vi "ros_test.vi"() -> ()   [LabVIEW 2015]
uses:
  <vilib>/Tufts CEEO ROS for LabVIEW Software/ROS/Code/Console/Servers/ServerSubs/TopicDef.ctl
  <vilib>/Tufts CEEO ROS for LabVIEW Software/ROS/Code/SubVIs/_ROSDirection.ctl
  <vilib>/Tufts CEEO ROS for LabVIEW Software/ROS/MessageParsing/std_msgs/subs/parse_i32_scalar.vi
panel:
  in  "stop":bool
  out "number":i32
  in  "node":string
  in  "Definitions":T1={"Topic"="/robot/head/command_head_nod", "Type"="std_msgs/Bool", "Action"=enum."Publisher", "Update (ms)"=1, "queue size"=1}
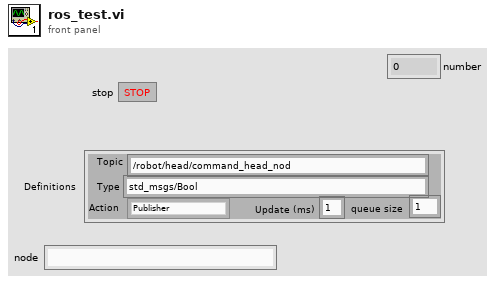
[diagram p1: front panel]
types:
  T1 = typedef "TopicDef.ctl" = cluster{"Topic":string, "Type":string, "Action":T2, "Update (ms)":u16, "queue size":u16}
  T2 = typedef "_ROSDirection.ctl" = enum16{"Node", "Publisher", "Subscriber", "ServiceClient", "ServiceProvider"}
  T3 = typedef "_ROSControl.ctl" = cluster{"topic port":u16, "Node":string, "topic":string, "type":string, "node port":u16, "error ":errorcluster, "Direction":T2, "Update (ms)":u16, "FIFO size":u16}
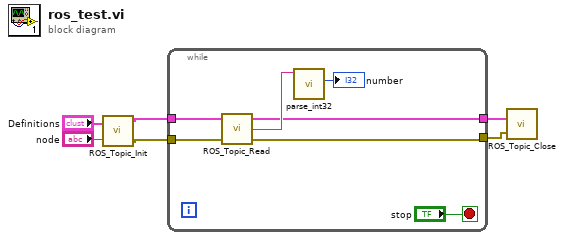
[diagram p0: block diagram]
diagram:
  n1 = call <vilib>:"ROS_Topic_Init.vi"("Definitions"="Definitions", "node"="node") -> ("ROS out"=w2:T3, "error out"=w1:errorcluster)  [unwired: 1 in]
  n2 = while {
    tunnel: [w10] -> w5
    tunnel: [w9] -> w6
    tunnel: w2 -> [w8]
    tunnel: w1 -> [w7]
    stop <- "stop" stop-if-true
    n3 = call <vilib>:"ROS_Topic_Read.vi"("error in (no error)"=w7, "ROS in"=w8) -> ("error out"=w9:errorcluster, "Reply"=w13:string, "ROS out"=w10:T3)  [unwired: 1 in]
    n4 = call-poly <vilib>:"parse_int32.vi"("msg in"=w13) -> ("number"=→"number":i32)  [unwired: 4 in, 2 out]
  }
  n5 = call <vilib>:"ROS_Topic_Close.vi"("error in"=w6, "ROS in"=w5) -> ()  [unwired: 2 in, 1 out]
